vi "Charger_Multi-Channel Init Buttons.vi"(6 "STOP refnum":refnum<vi>, 7 "RUN refnum":refnum<vi>, 8 "error in":errorcluster, 9 "PRINT refnum":refnum<vi>, 10 "VBAT refnum":refnum<vi>) -> (0 "error out":errorcluster)   [LabVIEW 2020]
doc: "This function initializes the RUN, STOP, and PRINT button \"Value\" and \"Disabled\" attributes."
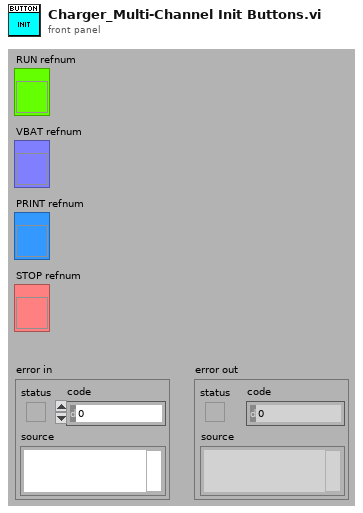
[diagram p1: front panel]
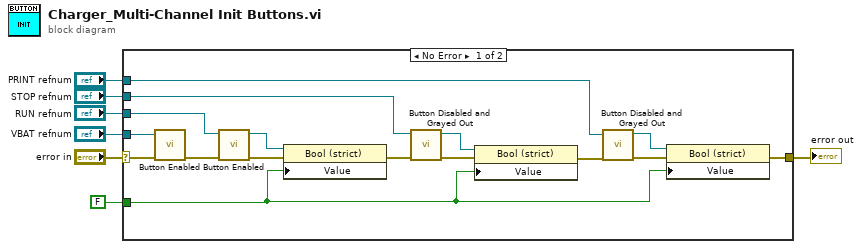
[diagram p0: block diagram]
diagram:
  n1 = case shown="No Error" "error in" {
    selector: "error in" -> [w10 w24]
    tunnel: "RUN refnum" -> [w21 _]
    tunnel: [w17 w24] -> w6
    tunnel: "STOP refnum" -> [w16 _]
    tunnel: "PRINT refnum" -> [w14 _]
    tunnel: FALSE ("Value") -> [w12 _]
    tunnel: "VBAT refnum" -> [w8 _]
    frame No Error {
      n2 = call "Button Enabled.vi"("error in"=w10, "button refnum"=w8) -> ("error out"=w9:errorcluster)  [unwired: 6 in, 1 out]
      n3 = call "Button Enabled.vi"("error in"=w9, "button refnum"=w21) -> ("error out"=w23:errorcluster, "button refnum dup"=w11:refnum<vi>)  [unwired: 6 in]
      n4 = property class="Bool (strict)"(reference=w11, error in=w23, "Value"=w12) -> (error out=w22:errorcluster)  [unwired: 1 out]
      n5 = call "Button Disabled and Grayed Out.vi"("error in"=w22, "button refnum"=w16) -> ("error out"=w20:errorcluster, "button refnum dup"=w15:refnum<vi>)  [unwired: 6 in]
      n6 = property class="Bool (strict)"(reference=w15, error in=w20, "Value"=w12) -> (error out=w19:errorcluster)  [unwired: 1 out]
      n7 = call "Button Disabled and Grayed Out.vi"("error in"=w19, "button refnum"=w14) -> ("error out"=w18:errorcluster, "button refnum dup"=w13:refnum<vi>)  [unwired: 6 in]
      n8 = property class="Bool (strict)"(reference=w13, error in=w18, "Value"=w12) -> (error out=w17:errorcluster)  [unwired: 1 out]
    }
    frame Error {
    }
  }
  "error out" <- w6
